vi "Test TCRS Temperature Stable if Heating Turned off.vi"(8 "error in (no error)":errorcluster, 11 "Thermal Chamber Response Simlator Test In":refnum<class "Thermal Chamber Response Simlator Test.lvclass">) -> (0 "error out":errorcluster, 3 "Thermal Chamber Response Simlator Test Out":refnum<class "Thermal Chamber Response Simlator Test.lvclass">)   [LabVIEW 2020, in "Thermal Chamber Response Simlator Test.lvclass"]
uses:
  Thermal Chamber Response Simlator Test.lvclass
  Thermal Chamber Response Simlator/Thermal Chamber Response Simlator.lvclass
  <vilib>/Asteme/LUnit/Test Case.lvclass
  C:/Program Files (x86)/National Instruments/LabVIEW 2020/vi.lib/Asteme/LUnit/Test Case.lvclass
  C:/Users/anton/Documents/GitHub/Triarc-Examples/Thermal Chamber/Thermal Chamber Response Simlator Test/Thermal Chamber Response Simlator Test.lvclass
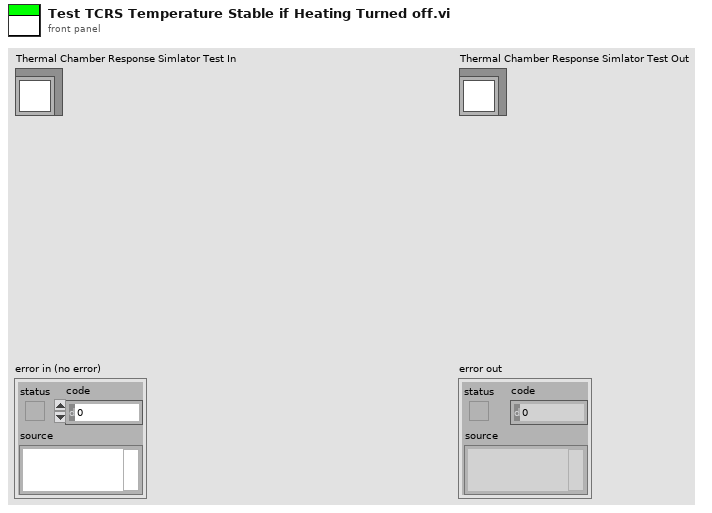
[diagram p1: front panel]
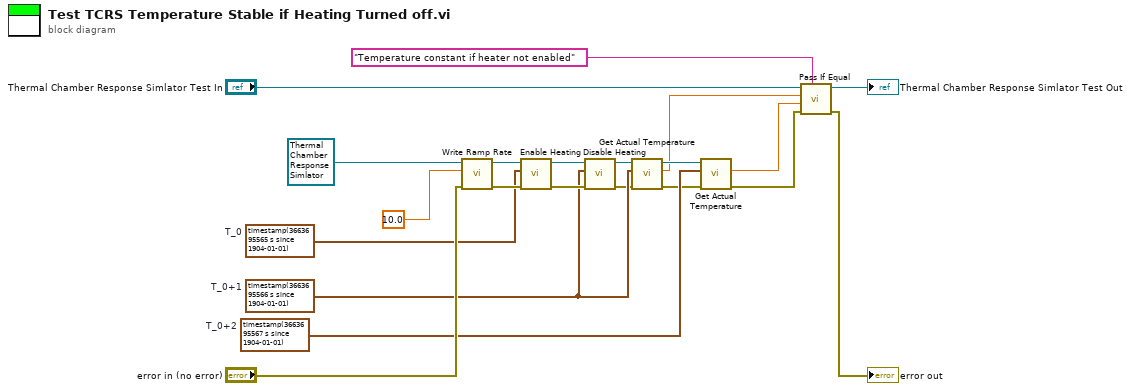
[diagram p0: block diagram]
diagram:
  w7 = timestamp(3663695567 s since 1904-01-01)  # T_0+2
  w5 = timestamp(3663695566 s since 1904-01-01)  # T_0+1
  w10 = timestamp(3663695565 s since 1904-01-01)  # T_0
  n1 = call "Write Ramp Rate.vi"("error in (no error)"="error in (no error)", "Ramp Rate [degC/s]"=10.0, "Thermal Chamber Response Simlator In"=refnum<class "Thermal Chamber Response Simlator.lvclass"> refnum ("Thermal Chamber Response Simlator.lvclass")) -> ("error out"=w19:errorcluster, "Thermal Chamber Response Simlator Out"=w12:refnum<class "Thermal Chamber Response Simlator.lvclass">)  [unwired: 7 in]
  n2 = call "Enable Heating.vi"("error in (no error)"=w19, "Start Time"=w10, "Thermal Chamber Response Simlator In"=w12) -> ("error out"=w8:errorcluster, "Thermal Chamber Response Simlator Out"=w9:refnum<class "Thermal Chamber Response Simlator.lvclass">)  [unwired: 7 in]
  n3 = call "Disable Heating.vi"("error in (no error)"=w8, "Start Time"=w5, "Thermal Chamber Response Simlator In"=w9) -> ("error out"=w3:errorcluster, "Thermal Chamber Response Simlator Out"=w6:refnum<class "Thermal Chamber Response Simlator.lvclass">)  [unwired: 7 in]
  n4 = call "Get Actual Temperature.vi"("error in (no error)"=w3, "Time Stamp"=w5, "Thermal Chamber Response Simlator In"=w6) -> ("error out"=w2:errorcluster, "Actual Temperature [degC]"=w1:dbl, "Thermal Chamber Response Simlator Out"=w4:refnum<class "Thermal Chamber Response Simlator.lvclass">)  [unwired: 6 in]
  n5 = call "Get Actual Temperature.vi"("error in (no error)"=w2, "Time Stamp"=w7, "Thermal Chamber Response Simlator In"=w4) -> ("error out"=w17:errorcluster, "Actual Temperature [degC]"=w16:dbl)  [unwired: 6 in, 1 out]
  n6 = call <vilib>:"Pass If Equal.vi"("Description"="Temperature constant if heater not enabled", "error in (no error)"=w17, "Actual"=w16, "Expected"=w1, "Test Case In"="Thermal Chamber Response Simlator Test In") -> ("error out"=→"error out":errorcluster, "Test Case Out"=→"Thermal Chamber Response Simlator Test Out":refnum<class "Thermal Chamber Response Simlator Test.lvclass">)  [unwired: 5 in]
